vi "svx_Pair Match.vi"(8 "error in (no error)":errorcluster, 11 "channel property":T1[](array[typedef]) {"probe angle [deg]" max=360; "direction" items=["CCW", "CW"]}) -> (0 "error out":errorcluster, 1 "Y":T1 {"probe angle [deg]" max=360; "direction" items=["CCW", "CW"]}, 2 "X":T1 {"probe angle [deg]" max=360; "direction" items=["CCW", "CW"]}, 3 "remaining":T1[](array[typedef]) {"probe angle [deg]" max=360; "direction" items=["CCW", "CW"]}, 4 "match index":i32, 5 "match?":bool)   [LabVIEW 2017]
uses:
  <vilib>/addons/Sound and Vibration/Order Analysis/Data Presentation/SubVIs/OAT MCM Channel Property.ctl
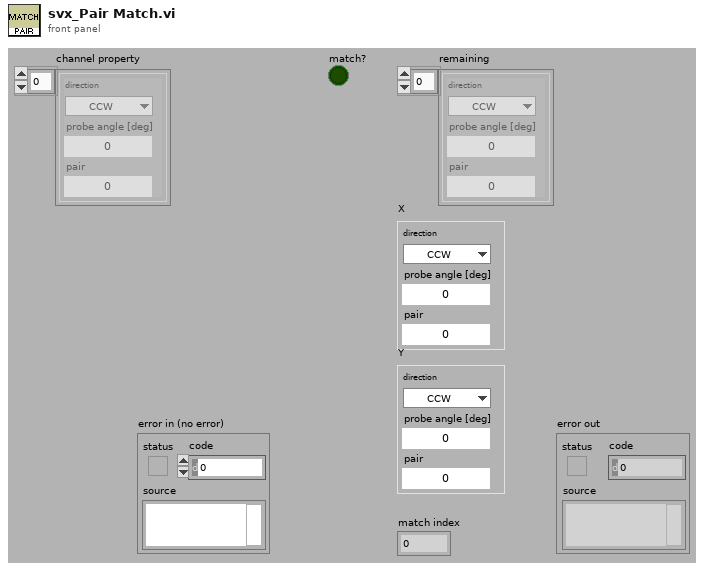
[diagram p1: front panel]
types:
  T1 = typedef "OAT MCM Channel Property.ctl" = cluster{"direction":u16, "probe angle [deg]":u16, "pair":u16}
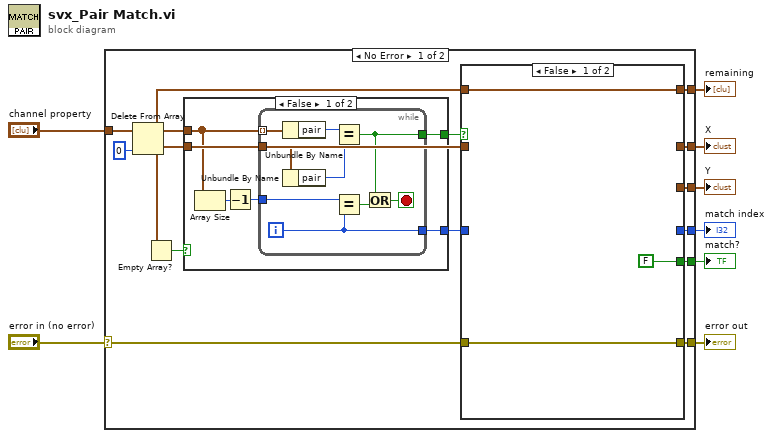
[diagram p0: block diagram]
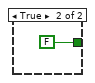
[diagram p2: hidden frame]
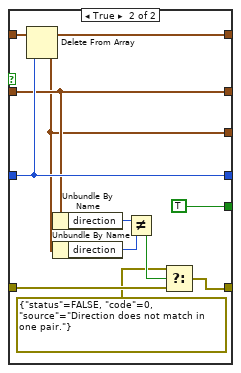
[diagram p3: hidden frame]
diagram:
  n1 = case shown="No Error" "error in (no error)" {
    selector: "error in (no error)" -> [w13 w54]
    tunnel: "channel property" -> [w22 _]
    tunnel: [w14 _] -> w2
    tunnel: [w20 _] -> w1
    tunnel: [w17 _] -> w8
    tunnel: [w16 _] -> w3
    tunnel: [w12 w54] -> w6
    tunnel: [w11 _] -> w5
    frame No Error {
      n2 = Delete From Array(array=w22, index=0) -> (deleted portion=w15:T1, array with subset deleted=w10:T1[])  [unwired: 1 in]
      n3 = Empty Array?(array=w10) -> (empty?=w9:bool)
      n4 = case shown="False" w9 {
        tunnel: [w26 _] -> w19
        tunnel: [w25 FALSE] -> w18
        tunnel: w15 -> [w24 _]
        tunnel: w10 -> [w23 _]
        frame False {
          n5 = Array Size(array=w23) -> (size(s)=w28:i32)
          n6 = Decrement(x=w28) -> (x-1=w27:i32)
          n7 = while {
            tunnel: w23 -> [w36] mode=indexing
            tunnel: w24 -> [w37]
            tunnel: w27 -> [w33]
            tunnel: [w30] -> w25
            tunnel: [w29] -> w26
            i -> [w29]
            stop <- w31 stop-if-true
            n8 = Unbundle By Name(w36) -> ("pair"=w35:u16)
            n9 = Unbundle By Name(w37) -> ("pair"=w34:u16)
            n10 = Equal?(x=w35, y=w34) -> (x = y?=w30:bool)
            n11 = Equal?(x=w33, y=w29) -> (x = y?=w32:bool)
            n12 = Or(x=w30, y=w32) -> (x .or. y?=w31:bool)
          }
        }
        frame True {
        }
      }
      n13 = case shown="False" w18 {
        tunnel: w10 -> [w41 w53]
        tunnel: [_ w49] -> w20
        tunnel: w19 -> [_ w52]
        tunnel: [_ w52] -> w17
        tunnel: [w41 w51] -> w16
        tunnel: w15 -> [_ w50]
        tunnel: [_ w50] -> w14
        tunnel: w13 -> [w40 w45]
        tunnel: [w40 w44] -> w12
        tunnel: [FALSE ("match?") TRUE ("match?")] -> w11
        frame False {
        }
        frame True {
          n14 = Delete From Array(array=w53, index=w52) -> (deleted portion=w49:T1, array with subset deleted=w51:T1[])  [unwired: 1 in]
          n15 = Unbundle By Name(w50) -> ("direction"=w48:u16)
          n16 = Unbundle By Name(w49) -> ("direction"=w47:u16)
          n17 = Not Equal?(x=w48, y=w47) -> (x != y?=w46:bool)
          n18 = Select(t=errorcluster {"status"=FALSE, "code"=0, "source"="Direction does not match in one pair."}, s=w46, f=w45) -> (s? t:f=w44:errorcluster)
        }
      }
    }
    frame Error {
    }
  }
  "match?" <- w5
  "match index" <- w8
  "error out" <- w6
  "remaining" <- w3
  "X" <- w2
  "Y" <- w1
